vi "svc_Convert Start and Stop to Start Index and Length.vi"(0 "f0":dbl format="%.2f", 5 "df":dbl format="%.2f", 7 "start frequency":dbl format="%.2f", 9 "stop frequency":dbl format="%.2f") -> (4 "start index":i32, 6 "band length":i32, 8 "f0 out":dbl format="%.2f", 10 "fmax out":dbl format="%.2f")   [LabVIEW 2017]
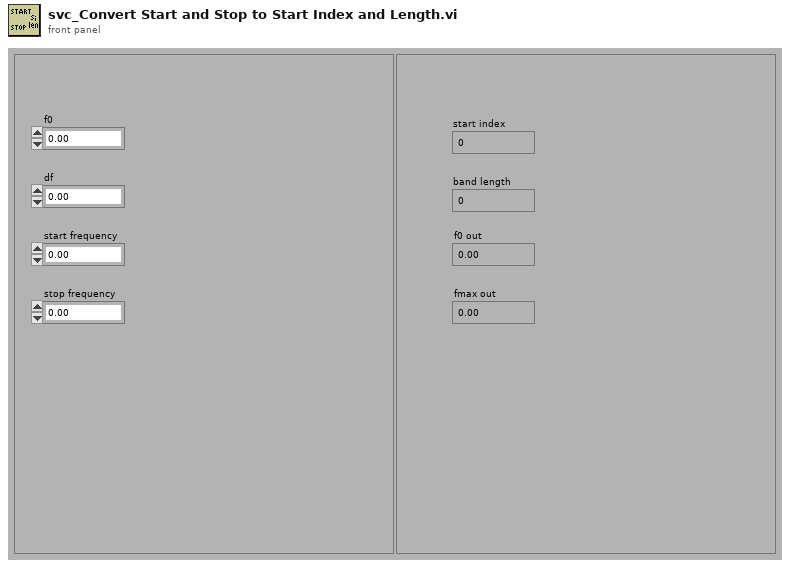
[diagram p1: front panel]
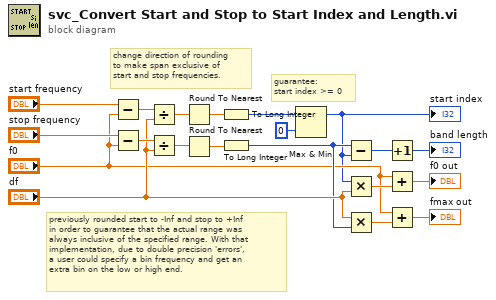
[diagram p0: block diagram]
diagram:
  # "guarantee:\nstart index >= 0"
  # "previously rounded start to -Inf and stop to +Inf\nin order to guarantee that the actual range was \nalways inclusive of the specified range. With that\nimplementation, due to double precision 'errors', \na user could specify a bin frequency and get an \nextra bin on the low or high end."
  # "change direction of rounding\nto make span exclusive of \nstart and stop frequencies."
  n1 = Subtract(x="start frequency", y="f0") -> (x-y=w14:dbl)
  n2 = Subtract(x="stop frequency", y="f0") -> (x-y=w12:dbl)
  n3 = Divide(x=w14, y="df") -> (x/y=w18:dbl)
  n4 = Divide(x=w12, y="df") -> (x/y=w19:dbl)
  n5 = Round To Nearest(number=w18) -> (nearest integer value=w17:dbl)
  n6 = Round To Nearest(number=w19) -> (nearest integer value=w20:dbl)
  n7 = To Long Integer(number=w17) -> (32bit integer=w2:i32)
  n8 = To Long Integer(number=w20) -> (32bit integer=w5:i32)
  n9 = Max & Min(x=w2, y=0) -> (max(x,y)=w1:i32)  [unwired: 1 out]
  "start index" <- w1
  n10 = Subtract(x=w5, y=w1) -> (x-y=w7:i32)
  n11 = Multiply(x=w1, y="df") -> (x*y=w11:dbl)
  n12 = Multiply(x="df", y=w5) -> (x*y=w10:dbl)
  n13 = Increment(x=w7) -> (x+1=→"band length":i32)
  n14 = Add(x="f0", y=w11) -> (x+y=→"f0 out":dbl)
  n15 = Add(x="f0", y=w10) -> (x+y=→"fmax out":dbl)
